vi "Programmatically Save Control Values 86 Updated 2016 09.vi"() -> ()   [LabVIEW 2012]
panel:
  in  "Numeric 2":dbl
  in  "STOP":bool
  in  "String":string="test"
  in  "Boolean 2":bool=TRUE
  in  "Numeric":dbl=35.0
  in  "Boolean":bool=TRUE
  in  "LOAD":bool
  in  "SAVE":bool
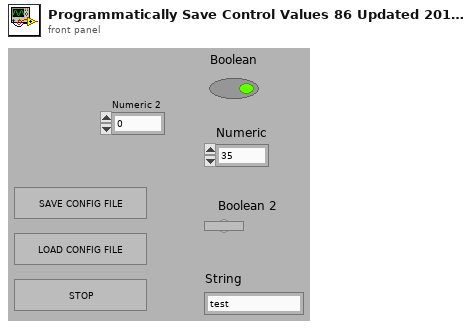
[diagram p1: front panel]
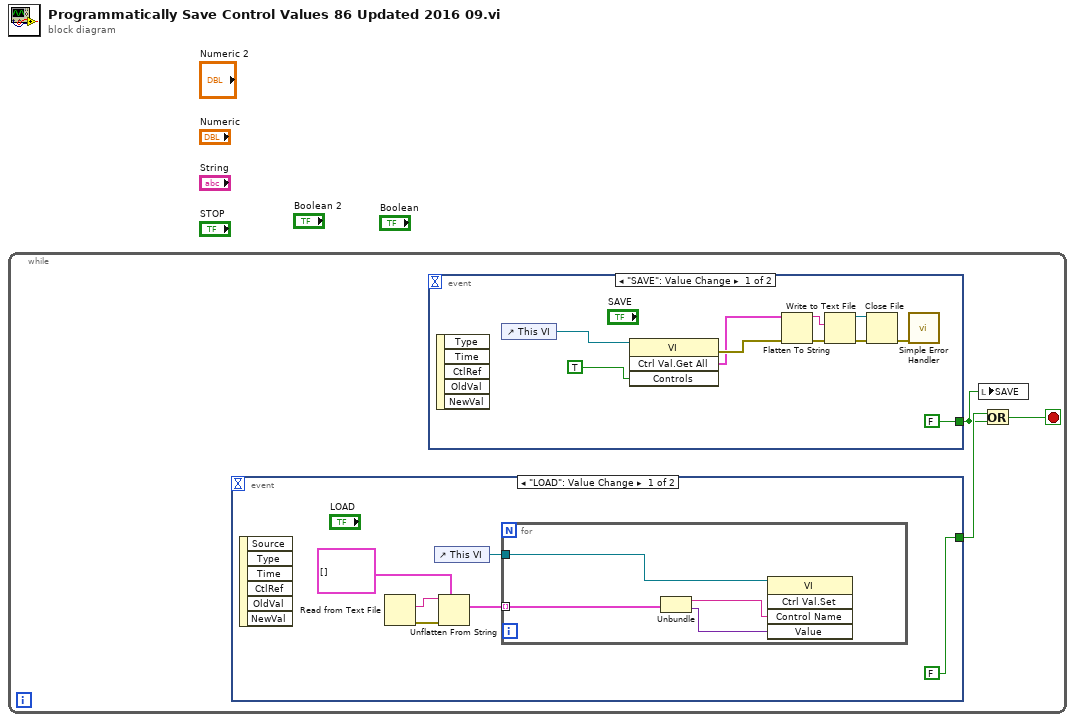
[diagram p0: block diagram]
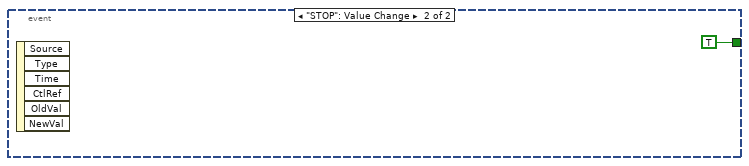
[diagram p2: hidden frame]
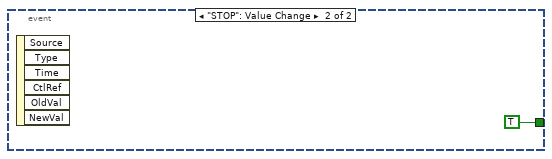
[diagram p3: hidden frame]
diagram:
  n1 = while {
    stop <- w2 stop-if-true
    n2 = event shown="[0] \"LOAD\": Value Change" {
      selector: _ -> [_ _]
      dyn-events: _ -> [_ _]
      timeout: _ -> [_ _]
      tunnel: [FALSE TRUE] -> w3
      event "LOAD": Value Change {
        n3 = event-data() -> ()  [unwired: 7 out]
        n4 = Read from Text File() -> (text=w7:string, error out=w6:errorcluster)  [unwired: 1 in, 5 out]
        n5 = control-ref of="This VI"() -> (w9:refnum<vi>)
        n6 = Unflatten From String(type=cluster{"Name":string, "Variant Data":variant}[] [] ("Control Value:Get All"), binary string=w7, error in (no error)=w6) -> (value=w8:cluster{"Name":string, "Variant Data":variant}[])  [unwired: 4 out]
        n7 = for {
          tunnel: w9 -> [w13]
          tunnel: w8 -> [w12] mode=indexing
          n8 = Unbundle(w12) -> ("Name"=w11:string, "Variant Data"=w10:variant)
          n9 = invoke class="VI" method="Ctrl Val.Set"(reference=w13, "Control Name"=w11, "Value"=w10) -> ()  [unwired: 2 in, 5 out]
        }
      }
      event "STOP": Value Change {
        n10 = event-data() -> ()  [unwired: 7 out]
      }
    }
    n11 = event shown="[0] \"SAVE\": Value Change" {
      selector: _ -> [_ _]
      dyn-events: _ -> [_ _]
      timeout: _ -> [_ _]
      tunnel: [FALSE TRUE] -> w1
      event "SAVE": Value Change {
        n12 = event-data() -> ()  [unwired: 6 out]
        n13 = control-ref of="This VI"() -> (w20:refnum<vi>)
        n14 = invoke class="VI" method="Ctrl Val.Get All"(reference=w20, "Controls"=TRUE) -> (error out=w22:errorcluster, "Get All Control Values Variant"=w15:cluster{"Name":string, "Variant Data":variant}[])  [unwired: 2 in, 2 out]
        n15 = Flatten To String(anything=w15, error in (no error)=w22) -> (data string=w23:string, error out=w21:errorcluster)  [unwired: 3 out]
        n16 = Write to Text File(text=w23, error in=w21) -> (refnum out=w18:refnum<file>, error out=w17:errorcluster)  [unwired: 3 out]
        n17 = Close File(refnum=w18, error in=w17) -> (error out=w19:errorcluster)  [unwired: 1 out]
        n18 = call <vilib>:"Simple Error Handler.vi"("error in (no error)"=w19) -> ()  [unwired: 1 in, 8 out]
      }
      event "STOP": Value Change {
        n19 = event-data() -> ()  [unwired: 7 out]
      }
    }
    n20 = local write "SAVE"(w1) -> ()
    n21 = Or(x=w3, y=w1) -> (x .or. y?=w2:bool)
  }
